vi "Find Tags CORE.vi"(11 "Index":string) -> (3 "Tags Front Matter":string)   [LabVIEW 2020]
doc: "This method loads the VIPMTag file on first call and uses it to find keywords in the Display Name and Description. When a keyword is found the cooresponding Tag is added to the Tag list."
uses:
  Libraries/Packages/Package_class/Package.lvclass/Package.ctl
  Libraries/Packages/Package Version_class/Package Version.lvclass/Package Version.ctl
  Libraries/Packages/Package Version_class/Read Author.vi
  Libraries/Packages/Package Version_class/Read Dependencies.vi
  Libraries/Packages/Package Version_class/Read Description.vi
  Libraries/Packages/Package Version_class/Read DisplayName.vi
  Libraries/Packages/Package Version_class/Read Name.vi
  Libraries/Packages/Package Version_class/Read Release Notes.vi
  Libraries/Packages/Package Version_class/Read RepoName.vi
  Libraries/Packages/Package Version_class/Read Vendor.vi
  Libraries/Packages/Package Version_class/Read Summary.vi
  Libraries/Packages/Package_class/Read DisplayName.vi
  Libraries/Packages/Package_class/Read Name.vi
  Libraries/Packages/Package_class/Read RepoName.vi
  Libraries/Packages/Package_class/Read Versions.vi
  <vilib>/Utility/file.llb/Read Delimited Spreadsheet (string).vi
  Libraries/Packages/Package Version_class/Package Version.lvclass
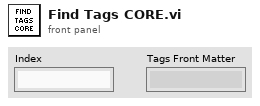
[diagram p1: front panel]
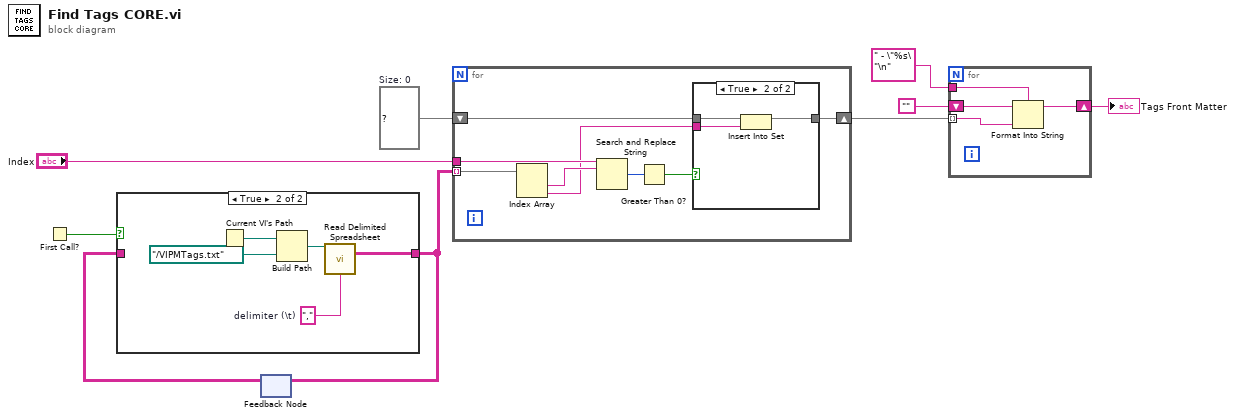
[diagram p0: block diagram]
diagram:
  w6 = set{string} {}  # Size: 0
  n1 = First Call?() -> (First Call?: T/F=w9:bool)
  n2 = feedback #1() -> (w7:string[][])  [unwired: 1 in]
  n3 = case shown="True" w9 {
    tunnel: [w10 w11] -> w8
    tunnel: w7 -> [w10 _]
    frame False {
    }
    frame True {
      w12 = ","  # delimiter (\t)
      n4 = Current VI's Path() -> (path=w15:path)
      n5 = Build Path(base path=w15, name or relative path=path "../VIPMTags.txt") -> (appended path=w13:path)
      n6 = call-poly <vilib>:"Read Delimited Spreadsheet.vi"("file path (dialog if empty)"=w13, "delimiter (\\t)"=w12) -> ("all rows"=w11:string[][])  [unwired: 8 in, 5 out]
    }
  }
  n7 = feedback-in #1(w8) -> ()
  n8 = for {
    tunnel: "Index" -> [w23]
    tunnel: w8 -> [w21] mode=indexing
    shift-right: [w17] -> w5
    shift-left: w6 -> [w16]
    n9 = Index Array(array=w21) -> (element #1=w20:string, element #2=w19:string)  [unwired: 2 in]
    n10 = Search and Replace String(input string=w23, search string=w20) -> (number of replacements=w22:i32)  [unwired: 6 in, 3 out]
    n11 = Greater Than 0?(x=w22) -> (x > 0?=w18:bool)
    n12 = case shown="True" w18 {
      tunnel: w19 -> [_ w27]
      tunnel: [w24 w26] -> w17
      tunnel: w16 -> [w24 w25]
      frame False {
      }
      frame True {
        n13 = Insert Into Set(10:w27, 11:w25) -> (3:w26:set{string})  [unwired: 1 out]
      }
    }
  }
  n14 = for {
    tunnel: w5 -> [w31] mode=indexing
    shift-right: [w29] -> w2
    shift-left: "" -> [w30]
    tunnel: " - \"%s\"\n" -> [w28]
    n15 = Format Into String(format string=w28, initial string=w30, w31) -> (resulting string=w29:string)  [unwired: 1 in, 1 out]
  }
  "Tags Front Matter" <- w2
